vi "Make Request.vi"(7 "Wait For Reply":bool, 8 "error in (no error)":errorcluster, 11 "Worker Queue":refnum<queue>) -> (0 "error out":errorcluster, 2 "Future":refnum<class "Future.lvclass">)   [LabVIEW 2017]
doc: "Make a request to the demo workers. \n\nSet \"Wait For Reply\" to use a synchronous wait for reply using a notifier."
uses:
  Command Queue Data.ctl
  Futures/Promise/Promise.lvclass
  Futures/Future/Future.lvclass
  Futures/Futures.lvlib
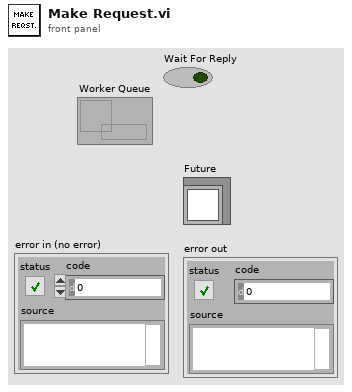
[diagram p1: front panel]
types:
  T1 = typedef "Command Queue Data.ctl" = cluster{"Promise":refnum<class "Promise.lvclass">, "notifier":refnum<notifier>}
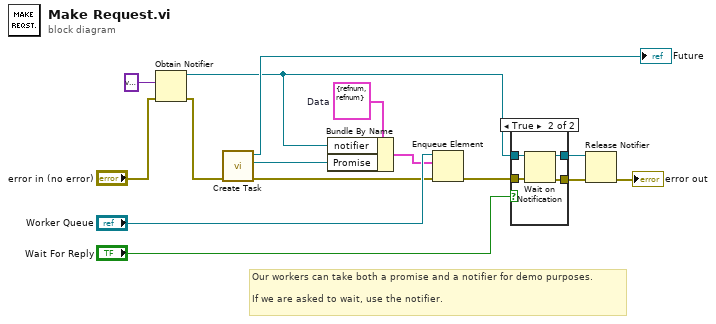
[diagram p0: block diagram]
diagram:
  w12 = T1 {"Promise"=refnum, "notifier"=refnum}  # Data
  # "Our workers can take both a promise and a notifier for demo purposes.\n\nIf we are asked to wait, use the notifier."
  n1 = Obtain Notifier(notification data type=variant ("Variant"), error in (no error)="error in (no error)") -> (notifier out=w3:refnum<notifier>, error out=w11:errorcluster)  [unwired: 2 in, 1 out]
  n2 = call "Create Task.vi"("error in (no error)"=w11) -> ("error out"=w8:errorcluster, "Promise out"=w10:refnum<class "Promise.lvclass">, "Future out"=→"Future":refnum<class "Future.lvclass">)  [unwired: 8 in]
  n3 = Bundle By Name(cluster=w12, "notifier"=w3, "Promise"=w10) -> (w9:T1)
  n4 = Enqueue Element(queue="Worker Queue", element=w9, error in (no error)=w8) -> (error out=w4:errorcluster)  [unwired: 1 in, 2 out]
  n5 = case shown="True" "Wait For Reply" {
    tunnel: [w16 w21] -> w6
    tunnel: [w17 w20] -> w5
    tunnel: w4 -> [w16 w19]
    tunnel: w3 -> [w17 w18]
    frame False {
    }
    frame True {
      n6 = Wait on Notification(notifier=w18, error in (no error)=w19) -> (notifier out=w20:refnum<notifier>, error out=w21:errorcluster)  [unwired: 2 in, 2 out]
    }
  }
  n7 = Release Notifier(notifier=w5, error in (no error)=w6) -> (error out=→"error out":errorcluster)  [unwired: 1 in, 2 out]
